vi "KundtsTube.vi"() -> ()   [LabVIEW 2015]
uses:
  <vilib>/imath/engines/lvmath2/RunTimeEngine/Managers/WorkSpace/UID Generator.vi
  <vilib>/imath/engines/lvmath2/RunTimeEngine/RunTimeType/NIMS_RunTimeType_From StrictType (excl LVString).vi
  <instcachedir>/0/NIMS_RunTimeType_From StrictType (excl LVString)_EB1C38A9BC5048DA9ABDA8F781E54D21.lvgen/NIMS_RunTimeType_From StrictType (excl LVString)_EB1C38A9BC5048DA9ABDA8F781E54D21_000.vi
  <vilib>/imath/engines/lvmath2/RunTimeEngine/LocalVariableDefStatement/MC_LocalVariableDefStatement_Display.vi
  <vilib>/imath/engines/lvmath2/RunTimeEngine/Managers/SymbolTable/Clear UID.vi
  <vilib>/imath/engines/lvmath2/RunTimeEngine/NodeEndStatement/NIMS_NodeEndStatement_Output.vi
  <instcachedir>/0/NIMS_NodeEndStatement_Output_53EC0D466D134D7ABD903AC30B43404B.lvgen/NIMS_NodeEndStatement_Output_53EC0D466D134D7ABD903AC30B43404B_009.vi
  <vilib>/imath/engines/lvmath2/RunTimeEngine/ErrorHandling/NIMS_Finalize Error.vi
  <vilib>/imath/engines/lvmath2/RunTimeEngine/IndexRead/NIMS M(S).vi
  <instcachedir>/0/NIMS M(S)_B826C018497E4940AE96BD27B540B6FB.lvgen/NIMS M(S)_B826C018497E4940AE96BD27B540B6FB_000.vi
  <vilib>/imathl/engines/lvmath/Functions/Error Handling/Create Error.vi
  <instcachedir>/0/NIMS_NodeEndStatement_Output_53EC0D466D134D7ABD903AC30B43404B.lvgen/NIMS_NodeEndStatement_Output_53EC0D466D134D7ABD903AC30B43404B_001.vi
  <vilib>/imath/engines/lvmath2/RunTimeEngine/Managers/SymbolTable/NIMS_WorkSpace.lvlib
panel:
  in  "Sample Parameters":T1={"Number of Samples"=100.0, "Sampling Rate (HZ)"=1000.0}
  in  "stop (T)":bool=TRUE
  in  "Amplitude":dbl=1.0
  out "Waveform":dynamicdata(graph)
  out "Gain Vs Frequency":cluster{dbl[], dbl[]}(graph)
  out "RMS Value":cdb
  in  "Tab Control":enum32{"Sweep", "Single"}(tab)
  in  "Dwell Time (ms)":dbl
  in  "Frequency (HZ)":dbl=1.0
  in  "Array Inputs":T2
  # "Sweeps frequencies from min. to \nmax., pausing for dwell time for\neach itiration"
  # "Plots waveform for a single \nfrequency"
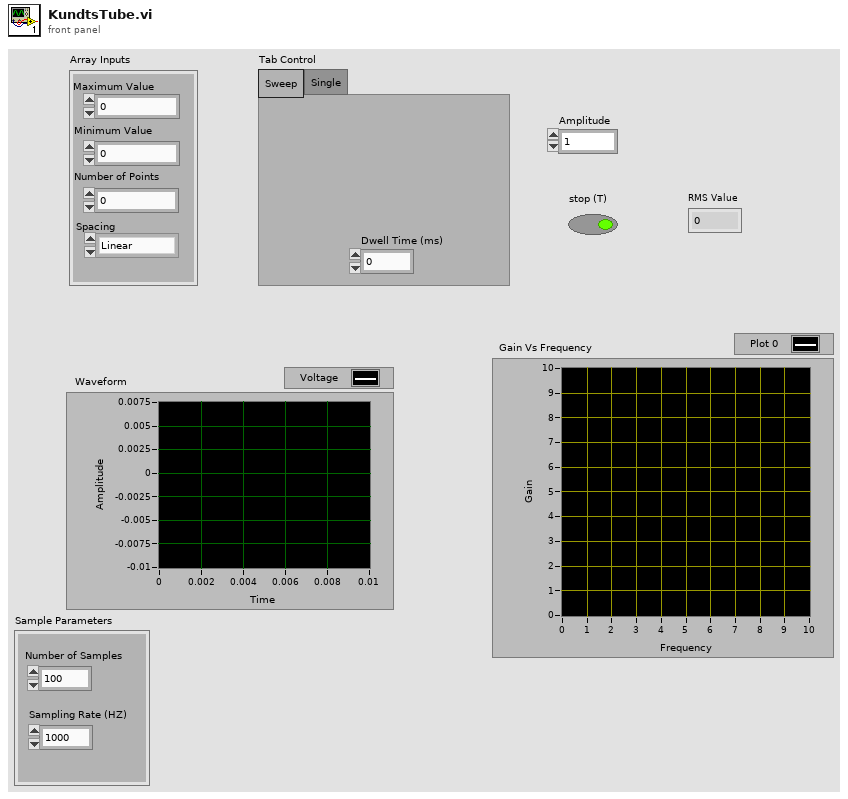
[diagram p1: front panel]
types:
  T1 = cluster{"Number of Samples":dbl, "Sampling Rate (HZ)":dbl}
  T2 = cluster{"Maximum Value":dbl, "Minimum Value":dbl, "Number of Points":dbl, "Spacing":enum16{"Linear", "Logarithmic"}}
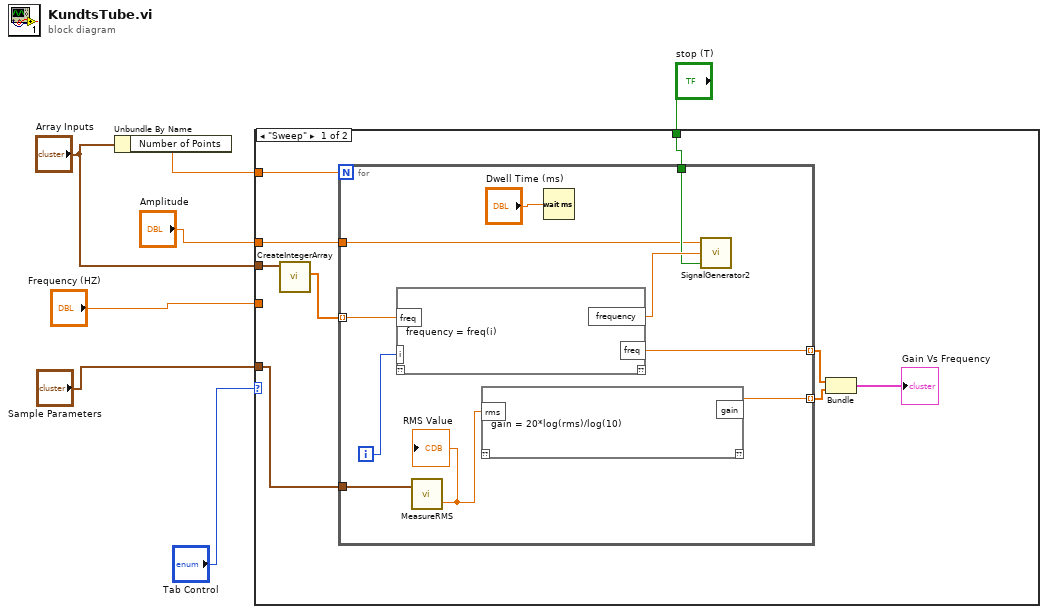
[diagram p0: block diagram]
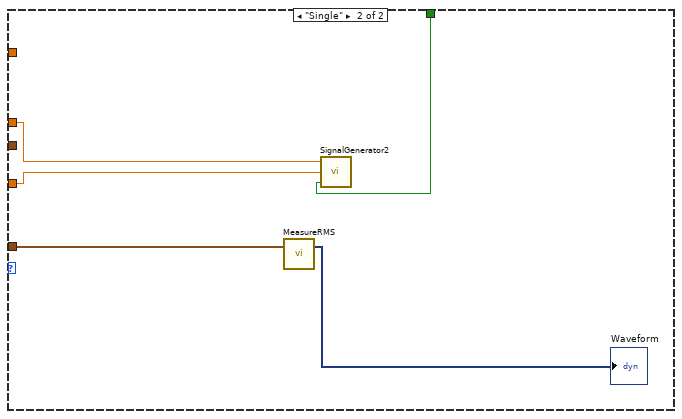
[diagram p2: hidden frame]
diagram:
  n1 = Unbundle By Name("Array Inputs") -> ("Number of Points"=w6:dbl)
  n2 = case shown="\"Sweep\"" "Tab Control" {
    tunnel: w6 -> [w16 _]
    tunnel: "Frequency (HZ)" -> [_ w126]
    tunnel: "Array Inputs" -> [w15 _]
    tunnel: "stop (T)" -> [w13 w125]
    tunnel: "Amplitude" -> [w12 w124]
    tunnel: "Sample Parameters" -> [w11 w123]
    frame "Sweep" {
      n3 = call "CreateIntegerArray.vi"("Array Inputs"=w15) -> ("vector"=w14:dbl[])  [unwired: 10 in]
      n4 = for {
        N: w16 -> [_]
        tunnel: w14 -> [w23] mode=indexing
        tunnel: [w22] -> w8 mode=indexing
        tunnel: [w21] -> w9 mode=indexing
        tunnel: w13 -> [w19]
        tunnel: w12 -> [w18]
        tunnel: w11 -> [w17]
        i -> [w25]
        n5 = mathscript code="frequency = freq(i)"("i"=w25, "freq"=w23) -> ("frequency"=w24:dbl, "freq"=w21:dbl)  [unwired: 1 in, 1 out]
        n6 = call "MeasureRMS.vi"("Sample Parameters"=w17) -> ("RMS Value"=w20:cdb)  [unwired: 1 in, 1 out]
        "RMS Value" <- w20
        n7 = mathscript code="gain = 20*log(rms)/log(10)"("rms"=w20) -> ("gain"=w22:cdb)  [unwired: 1 in, 1 out]
        n8 = Wait (ms)(milliseconds to wait="Dwell Time (ms)") -> ()  [unwired: 1 out]
        n9 = call "SignalGenerator2.vi"("stop (T)"=w19, "Frequency"=w24, "Amplitude"=w18) -> ()  [unwired: 1 in]
      }
      n10 = Bundle(w9, w8) -> (→"Gain Vs Frequency":cluster{dbl[], cdb[]})  [unwired: 1 in]
    }
    frame "Single" {
      n11 = call "MeasureRMS.vi"("Sample Parameters"=w123) -> ("Analog Signal Input Graph"=→"Waveform":dynamicdata)  [unwired: 1 in, 1 out]
      n12 = call "SignalGenerator2.vi"("stop (T)"=w125, "Frequency"=w126, "Amplitude"=w124) -> ()  [unwired: 1 in]
    }
  }
